vi "Itertools_Example.vi"() -> ()   [LabVIEW 2017]
uses:
  <userlib>/_OpenG.lib/array/array.llb/Filter 1D Array with Scalar (String)__ogtk.vi
  <vilib>/gmath/NI_Gmath.lvlib
panel:
  out "Itertools final arbitrary data-type list":string[](array[string])
  out "NI Cartesian product string list":string[](array[string])
  out "Itertools final string list":string[](array[string])
  out "NI Cartesian product path list":path[](array[path])
  out "NI Cartesian product string 2D-Array":string[][](array[string])
  out "Cartesian Product of Lists":i32[][](array[numeric])
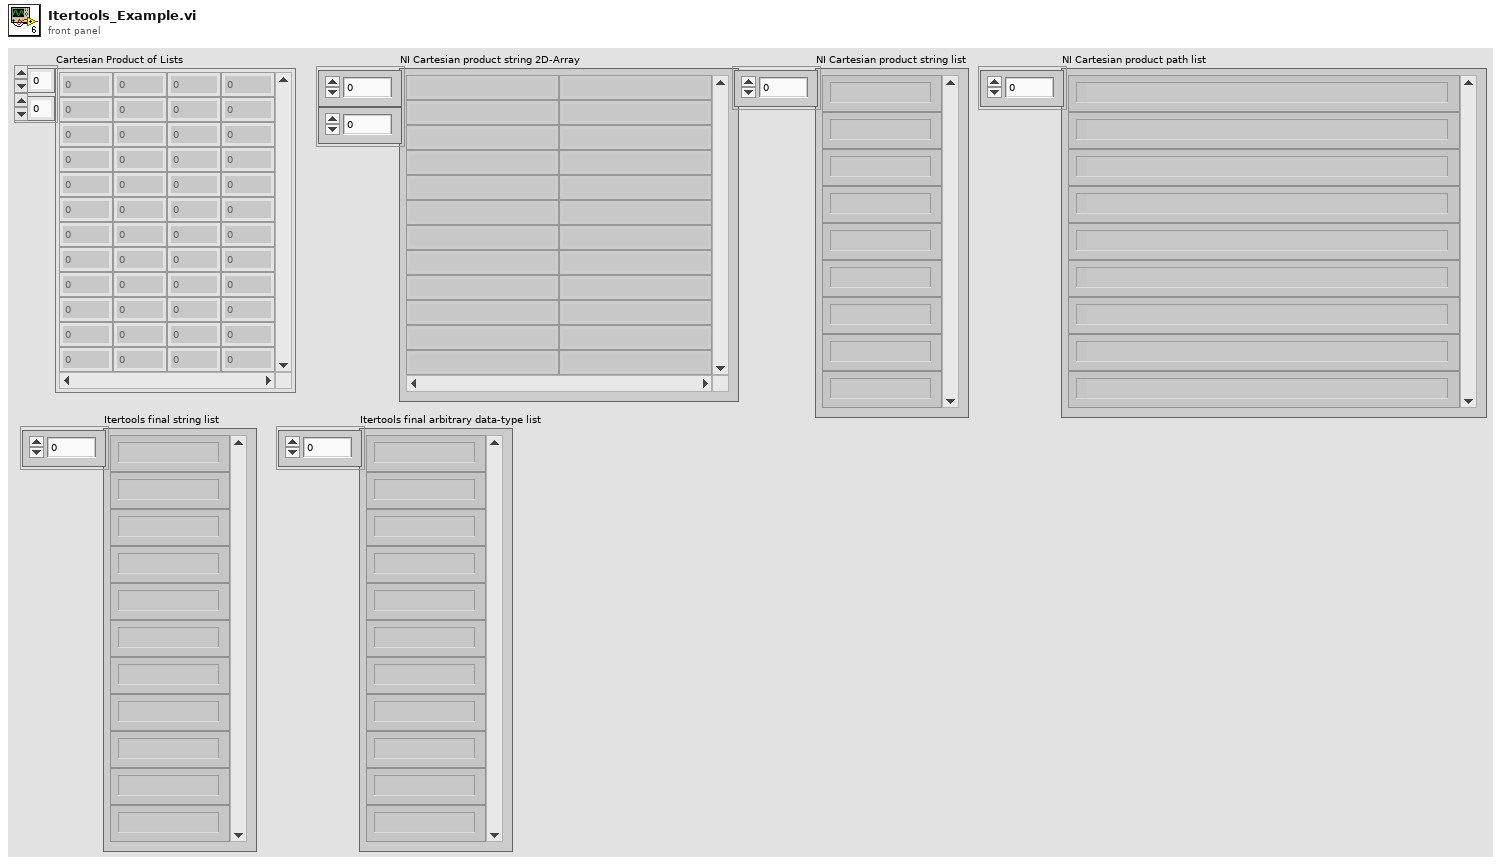
[diagram p1: front panel]
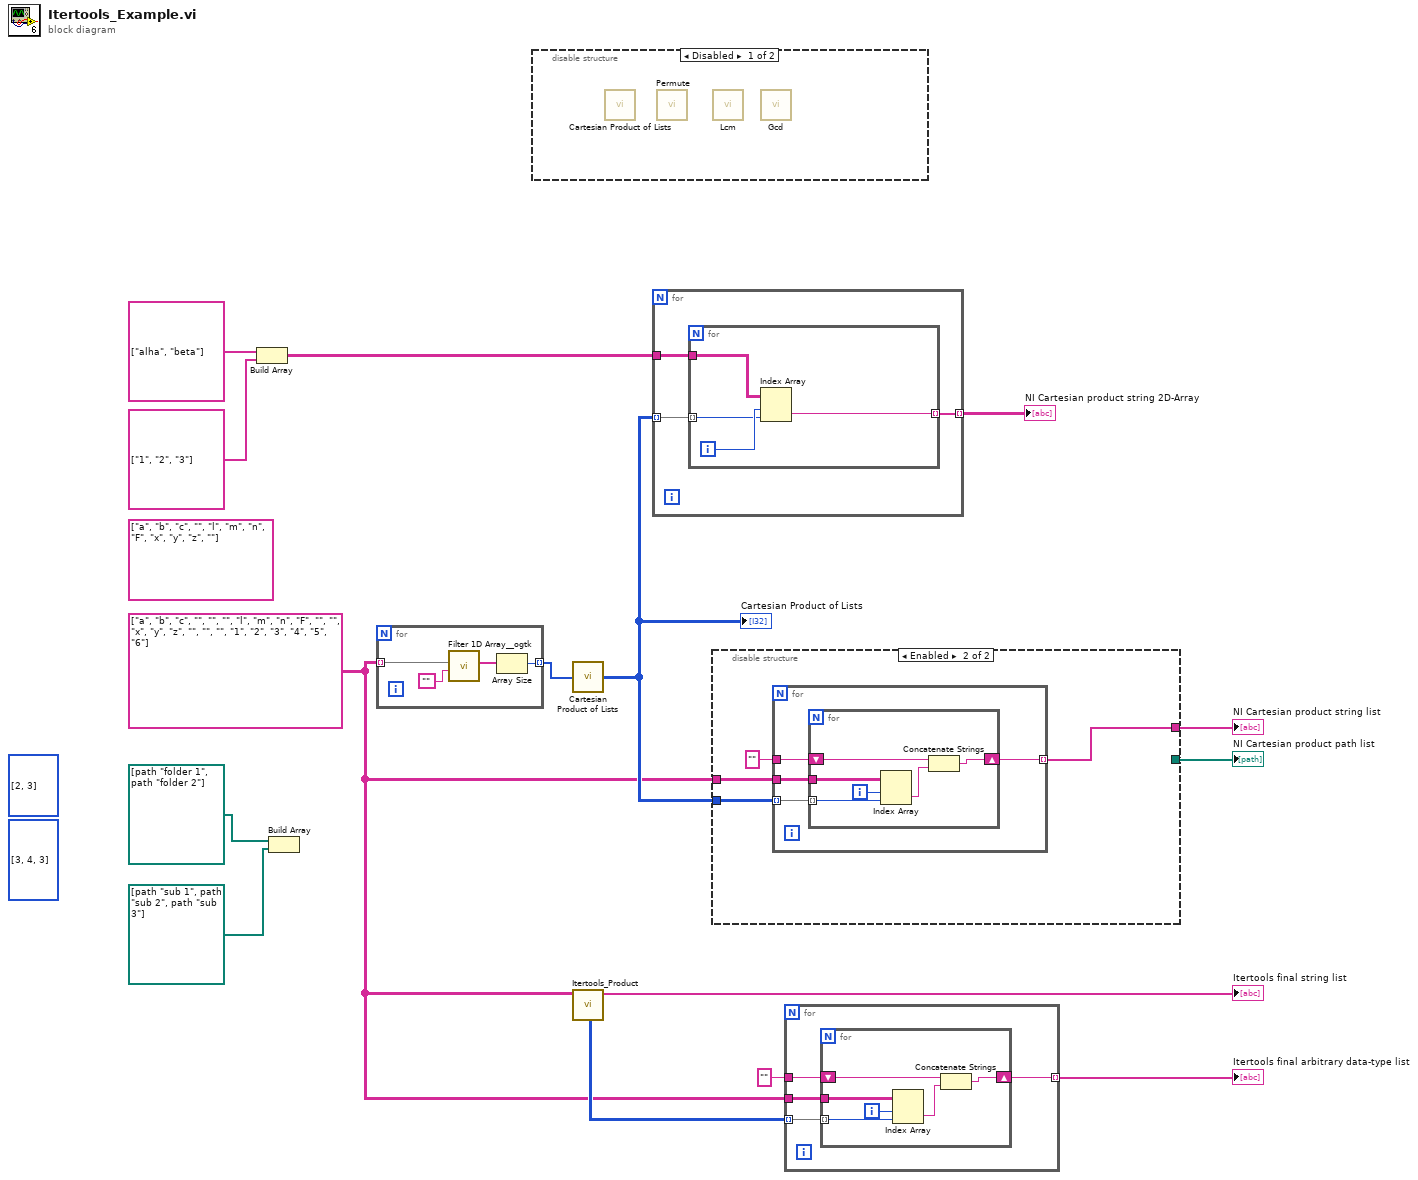
[diagram p0: block diagram]
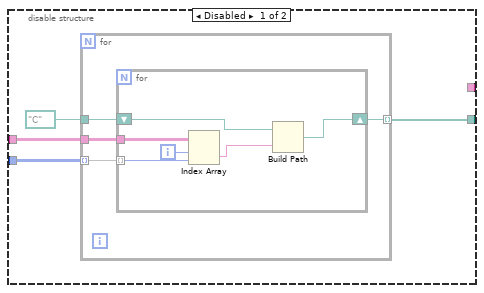
[diagram p2: hidden frame]
diagram:
  (unwired) string[][] [["a", "b", "c", ""], ["l", "m", "n", "F"], ["x", "y", "z", ""]] ("Array String")
  (unwired) i32[] [2, 3] ("Number of Elements in Each List")
  w2 = string[][] [["a", "b", "c", "", "", ""], ["l", "m", "n", "F", "", ""], ["x", "y", "z", "", "", ""], ["1", "2", "3", "4", "5", "6"]] ("Array String")
  (unwired) i32[] [3, 4, 3] ("Number of Elements in Each List")
  n1 = Build Array(string[] ["alha", "beta"], string[] ["1", "2", "3"]) -> (w14:string[][])
  n2 = Build Array(path[] [path "folder 1", path "folder 2"], path[] [path "sub 1", path "sub 2", path "sub 3"]) -> ()  [unwired: 1 out]
  n3 = for {
    tunnel: w2 -> [w19] mode=indexing
    tunnel: [w16] -> w7 mode=indexing
    n4 = call-poly <userlib>:"Filter 1D Array__ogtk.vi"("items to filter"="", "array"=w19) -> ("filtered array"=w17:string[])  [unwired: 4 in, 1 out]
    n5 = Array Size(array=w17) -> (size(s)=w16:i32)
  }
  n6 = disable-structure shown="Disabled" {
    frame Disabled {
      n7 = call <vilib>:"Cartesian Product of Lists.vi"() -> ()  [unwired: 1 in, 1 out]
      n8 = call <vilib>:"Permute.vi"() -> ()  [unwired: 2 in, 1 out]
      n9 = call <vilib>:"Lcm.vi"() -> ()  [unwired: 2 in, 1 out]
      n10 = call <vilib>:"Gcd.vi"() -> ()  [unwired: 2 in, 1 out]
    }
    frame Enabled {
    }
  }
  n11 = call <vilib>:"Cartesian Product of Lists.vi"("Number of Elements in Each List"=w7) -> ("Cartesian Product of Lists"=w12:i32[][])
  "Cartesian Product of Lists" <- w12
  n12 = call "Itertools_Product.vi"("Array List (in)"=w2) -> ("Product Indicies Array (Out)"=w5:i32[][], "Product Flattened String-Array (Out)"=→"Itertools final string list":string[])  [unwired: 8 in, 1 out]
  n13 = for {
    tunnel: w12 -> [w22] mode=indexing
    tunnel: w14 -> [w21]
    tunnel: [w20] -> w13 mode=indexing
    n14 = for {
      tunnel: w22 -> [w24] mode=indexing
      tunnel: w21 -> [w26]
      tunnel: [w23] -> w20 mode=indexing
      i -> [w25]
      n15 = Index Array(array=w26, index (row)=w25, index (col)=w24) -> (element=w23:string)
    }
  }
  "NI Cartesian product string 2D-Array" <- w13
  n16 = disable-structure shown="Enabled" {
    disable-tunnel: w12 -> [w30 w43]
    disable-tunnel: w2 -> [w29 w44]
    disable-tunnel: [w27 _] -> w9
    disable-tunnel: [_ w41] -> w8
    frame Disabled {
      n17 = for {
        tunnel: w30 -> [w34] mode=indexing
        tunnel: w29 -> [w33]
        tunnel: path "C:/" -> [w32]
        tunnel: [w31] -> w27 mode=indexing
        n18 = for {
          tunnel: w34 -> [w39] mode=indexing
          tunnel: w33 -> [w38]
          shift-right: [w35] -> w31
          shift-left: w32 -> [w37]
          i -> [w40]
          n19 = Index Array(array=w38, index (row)=w40, index (col)=w39) -> (element=w36:string)
          n20 = Build Path(base path=w37, name or relative path=w36) -> (appended path=w35:path)
        }
      }
    }
    frame Enabled {
      n21 = for {
        tunnel: w43 -> [w48] mode=indexing
        tunnel: w44 -> [w47]
        tunnel: "" ("String") -> [w46]
        tunnel: [w45] -> w41 mode=indexing
        n22 = for {
          tunnel: w48 -> [w53] mode=indexing
          tunnel: w47 -> [w52]
          shift-right: [w49] -> w45
          shift-left: w46 -> [w50]
          i -> [w54]
          n23 = Index Array(array=w52, index (row)=w54, index (col)=w53) -> (element=w51:string)
          n24 = Concatenate Strings(w50, w51) -> (w49:string)
        }
      }
    }
  }
  "NI Cartesian product path list" <- w9
  "NI Cartesian product string list" <- w8
  n25 = for {
    tunnel: w5 -> [w58] mode=indexing
    tunnel: "" ("String") -> [w57]
    tunnel: [w56] -> w1 mode=indexing
    tunnel: w2 -> [w55]
    n26 = for {
      tunnel: w58 -> [w63] mode=indexing
      shift-right: [w61] -> w56
      shift-left: w57 -> [w62]
      tunnel: w55 -> [w60]
      i -> [w64]
      n27 = Index Array(array=w60, index (row)=w64, index (col)=w63) -> (element=w59:string)
      n28 = Concatenate Strings(w62, w59) -> (w61:string)
    }
  }
  "Itertools final arbitrary data-type list" <- w1
